vi "rotate-part1.vi"(10 "Angle":i32, 11 "SceneObject输入":refnum<vi>) -> ()   [LabVIEW 2013]
uses:
  <vilib>/picture/3D Picture Control/NI_3D Picture Control.lvlib
panel:
  # "这是一个可重入的VI"
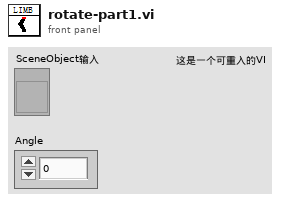
[diagram p1: front panel]
types:
  T1 = cluster{"zuoqian1":refnum<vi>, "zuoqian2":refnum<vi>, "zuoqian3":refnum<vi>}
  T2 = cluster{"youhou1":refnum<vi>, "youhou2":refnum<vi>, "youhou3":refnum<vi>}
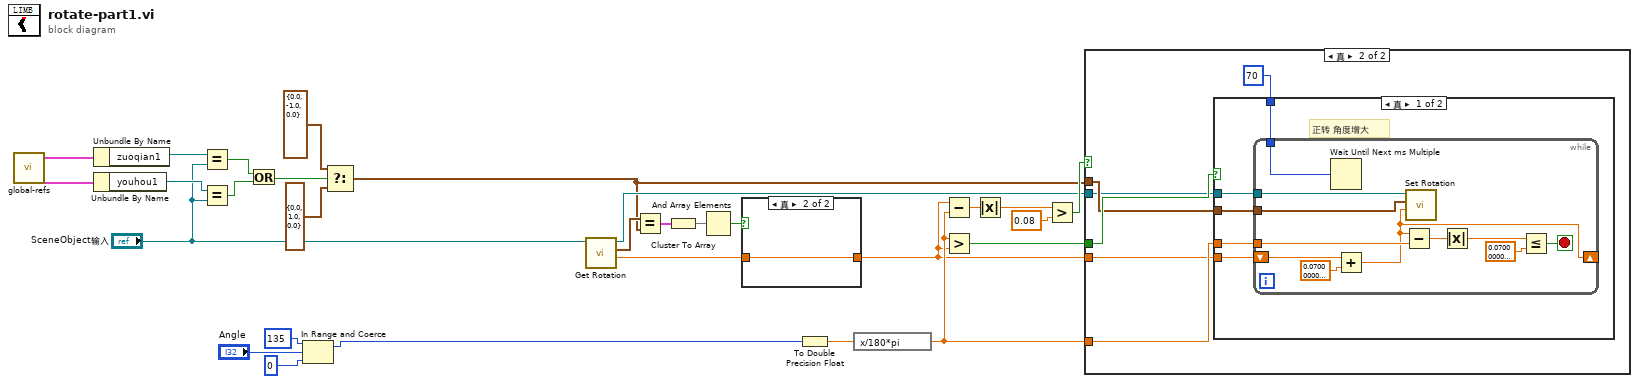
[diagram p0: block diagram]
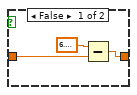
[diagram p2: hidden frame]
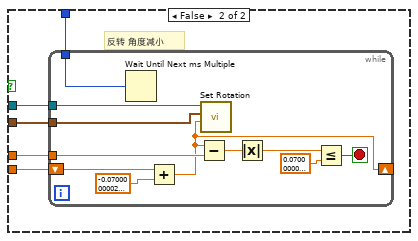
[diagram p4: hidden frame]
diagram:
  n1 = call "global-refs.vi"() -> ("ZuoQianRef"=w15:T1, "YouHouRef"=w14:T2)  [unwired: 10 in, 4 out]
  n2 = Unbundle By Name(w15) -> ("zuoqian1"=w12:refnum<vi>)
  n3 = Unbundle By Name(w14) -> ("youhou1"=w13:refnum<vi>)
  n4 = Equal?(x=w12, y="SceneObject输入") -> (x = y?=w9:bool)
  n5 = Equal?(x=w13, y="SceneObject输入") -> (x = y?=w10:bool)
  n6 = Or(x=w9, y=w10) -> (x .or. y?=w8:bool)
  n7 = In Range and Coerce(upper limit=135 ("上限"), x="Angle", lower limit=0 ("下限")) -> (coerced(x)=w1:i32)  [unwired: 1 out]
  n8 = Select(t=cluster{"X":sgl, "Y":sgl, "Z":sgl} {"X"=0.0, "Y"=-1.0, "Z"=0.0} ("Axis"), s=w8, f=cluster{"X":sgl, "Y":sgl, "Z":sgl} {"X"=0.0, "Y"=1.0, "Z"=0.0} ("Axis")) -> (s? t:f=w6:cluster{"X":sgl, "Y":sgl, "Z":sgl})
  n9 = call <vilib>:"Get Rotation.vi"("Scene Object"="SceneObject输入") -> ("Angle"=w17:sgl, "Axis"=w21:cluster{"X":sgl, "Y":sgl, "Z":sgl}, "Scene Object"=w22:refnum<vi>)  [unwired: 7 in, 1 out]
  n10 = Equal?(x=w21, y=w6) -> (x = y?=w20:cluster{"X":bool, "Y":bool, "Z":bool})
  n11 = Cluster To Array(cluster=w20) -> (array=w19:bool[])
  n12 = And Array Elements(Boolean array=w19) -> (logical AND=w18:bool)
  n13 = case shown="真" w18 {
    tunnel: w17 -> [w31 w33]
    tunnel: [w30 w33] -> w16
    frame False {
      n14 = Subtract(x=6.283185307179586, y=w31) -> (x-y=w30:dbl)
    }
    frame True {
    }
  }
  n15 = To Double Precision Float(number=w1) -> (double precision float=w29:dbl)
  n16 = expression code="x/180*pi"(w29) -> (w26:dbl)
  n17 = Subtract(x=w16, y=w26) -> (x-y=w27:dbl)
  n18 = Greater?(x=w26, y=w16) -> (0:w28:bool)
  n19 = Absolute Value(x=w27) -> (abs(x)=w25:dbl)
  n20 = Greater?(x=w25, y=0.08) -> (0:w23:bool)
  n21 = case shown="真" w23 {
    tunnel: w28 -> [_ w39]
    tunnel: w6 -> [_ w38]
    tunnel: w26 -> [_ w37]
    tunnel: w22 -> [_ w36]
    tunnel: w16 -> [_ w35]
    frame False {
      # "实际转角与设定转角差值很小, 不用转动"
    }
    frame True {
      n22 = case shown="真" w39 {
        tunnel: w38 -> [w41 w57]
        tunnel: w37 -> [w42 w58]
        tunnel: w36 -> [w44 w60]
        tunnel: w35 -> [w43 w59]
        tunnel: u32 70 ("毫秒倍数") -> [w40 w56]
        frame True {
          # "正转 角度增大"
          n23 = while {
            tunnel: w44 -> [w55]
            shift-right: [w46] -> _
            shift-left: w43 -> [w54]
            tunnel: w42 -> [w51]
            tunnel: w41 -> [w53]
            tunnel: w40 -> [w45]
            stop <- w47 stop-if-true
            n24 = Wait Until Next ms Multiple(millisecond multiple=w45) -> ()  [unwired: 1 out]
            n25 = Add(x=w54, y=sgl 0.07) -> (x+y=w46:dbl)
            n26 = Subtract(x=w46, y=w51) -> (x-y=w50:dbl)
            n27 = call <vilib>:"Set Rotation.vi"("Angle"=w46, "Axis"=w53, "Scene Object"=w55) -> ()  [unwired: 7 in, 2 out]
            n28 = Absolute Value(x=w50) -> (abs(x)=w49:dbl)
            n29 = Less Or Equal?(x=w49, y=sgl 0.07) -> (x <= y?=w47:bool)
          }
        }
        frame False {
          # "反转 角度减小"
          n30 = while {
            tunnel: w60 -> [w71]
            shift-right: [w62] -> _
            shift-left: w59 -> [w70]
            tunnel: w58 -> [w67]
            tunnel: w57 -> [w69]
            tunnel: w56 -> [w61]
            stop <- w63 stop-if-true
            n31 = Wait Until Next ms Multiple(millisecond multiple=w61) -> ()  [unwired: 1 out]
            n32 = Add(x=w70, y=sgl -0.07) -> (x+y=w62:dbl)
            n33 = Subtract(x=w62, y=w67) -> (x-y=w66:dbl)
            n34 = call <vilib>:"Set Rotation.vi"("Angle"=w62, "Axis"=w69, "Scene Object"=w71) -> ()  [unwired: 7 in, 2 out]
            n35 = Absolute Value(x=w66) -> (abs(x)=w65:dbl)
            n36 = Less Or Equal?(x=w65, y=sgl 0.07) -> (x <= y?=w63:bool)
          }
        }
      }
    }
  }
